vi "Get Signal From SVG.vi"(11 "file path (use dialog)":path) -> (3 "Signal":cdb[](array[numeric]))   [LabVIEW 2020]
panel:
  out "text":string
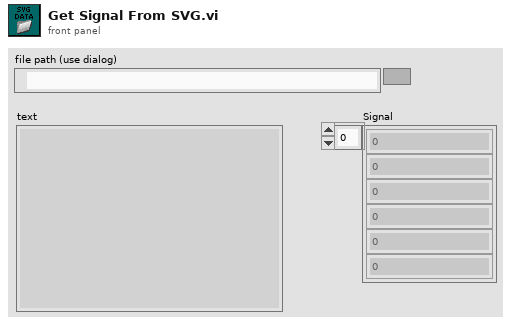
[diagram p1: front panel]
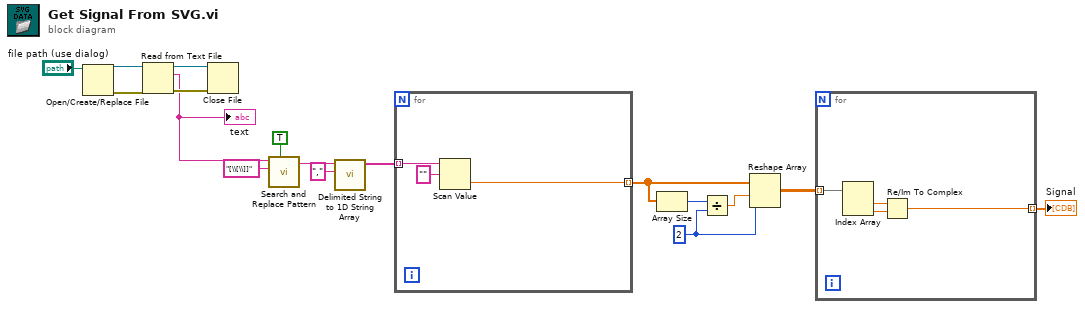
[diagram p0: block diagram]
diagram:
  w2 = 2 ("dimension size")
  n1 = Open/Create/Replace File(file path (use dialog)="file path (use dialog)") -> (refnum out=w15:refnum<file>, error out=w14:errorcluster)  [unwired: 5 in, 1 out]
  n2 = Read from Text File(file (use dialog)=w15, error in=w14) -> (refnum out=w16:refnum<file>, text=w12:string, error out=w17:errorcluster)  [unwired: 2 in, 1 out]
  "text" <- w12
  n3 = Close File(refnum=w16, error in=w17) -> ()  [unwired: 2 out]
  n4 = call <vilib>:"Search and Replace Pattern.vi"("string"=w12, "regular expression (\"\")"="[\\[\\]]" ("regular expression (\"\")"), "replace all? (F)"=TRUE) -> ("result string"=w9:string)  [unwired: 2 in, 1 out]
  n5 = call <vilib>:"Delimited String to 1D String Array.vi"("delimiter"=",", "delimited string"=w9) -> ("string array"=w7:string[])  [unwired: 9 in]
  n6 = for {
    tunnel: w7 -> [w20] mode=indexing
    tunnel: [w19] -> w4 mode=indexing
    n7 = Scan Value(string=w20, format string="") -> (value=w19:dbl)  [unwired: 1 in, 1 out]
  }
  n8 = Array Size(array=w4) -> (size(s)=w3:i32)
  n9 = Divide(x=w3, y=w2) -> (x/y=w1:dbl)
  n10 = Reshape Array(w4, w1, w2) -> (w6:dbl[][])
  n11 = for {
    tunnel: w6 -> [w24] mode=indexing
    tunnel: [w21] -> w5 mode=indexing
    n12 = Index Array(array=w24) -> (element #1=w22:dbl, element #2=w23:dbl)  [unwired: 2 in]
    n13 = Re/Im To Complex(1:w23, 2:w22) -> (0:w21:cdb)
  }
  "Signal" <- w5
